vi "Kp报文计算公式.vi"(1 "Kp":dbl(slide) scale=0.0..500.0) -> (0 "Kp报文":string)   [LabVIEW 2023]
panel:
  in  "选项卡控件":enum32{"选项卡 1", "选项卡 2"}(tab)
  out "16进制字符串":string
  out "十进制数":i32
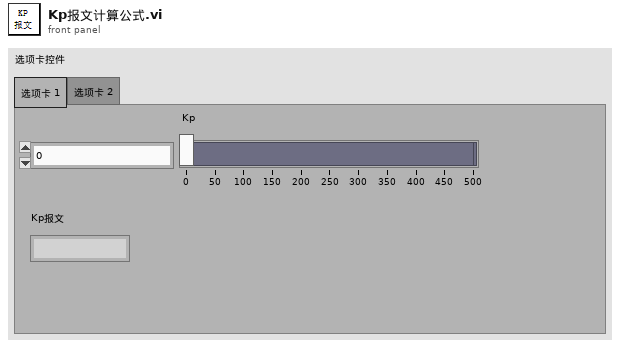
[diagram p1: front panel]
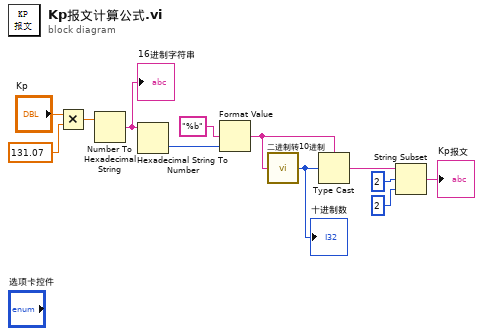
[diagram p0: block diagram]
diagram:
  n1 = Multiply(x="Kp", y=131.07) -> (x*y=w1:dbl)
  n2 = Number To Hexadecimal String(2:w1) -> (0:w7:string)  [unwired: 1 in]
  "16进制字符串" <- w7
  n3 = Hexadecimal String To Number(string=w7) -> (number=w10:u32)  [unwired: 2 in, 1 out]
  n4 = Format Value(format string="%b" ("格式字符串"), value (0)=w10) -> (output string=w8:string)  [unwired: 1 in]
  n5 = call "二进制转10进制.vi"("字符串"=w8) -> ("十进制数"=w9:i32)
  "十进制数" <- w9
  n6 = Type Cast(type=w8, x=w9) -> (*(type *) &x=w6:string)
  n7 = String Subset(string=w6, offset (0)=2 ("偏移量(0)"), length (rest)=2 ("长度（剩余）")) -> (substring=→"Kp报文":string)
